vi "Global 1.vi"() -> ()   [LabVIEW 2015]
panel:
  in  "String":string
  in  "Boolean":bool
  in  "Numeric":dbl
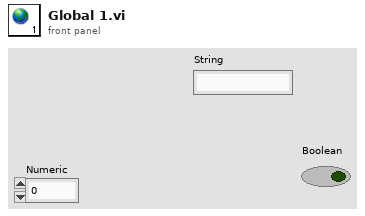
[diagram p1: front panel]
diagram:
